vi "Read SubVIs.vi"(9 "Diagram in":refnum<class "Diagram.lvclass">) -> (3 "Diagram out":refnum<class "Diagram.lvclass">, 4 "SubVIs":refnum<class "SubVI.lvclass">[](array[class]))   [LabVIEW 2014, in "Diagram.lvclass"]
uses:
  Diagram.lvclass
  SubVI/SubVI.lvclass
  Diagram.lvclass/Diagram.ctl
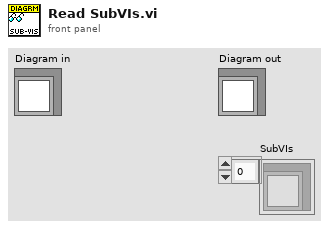
[diagram p1: front panel]
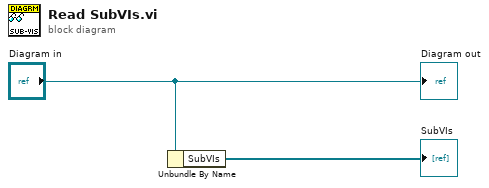
[diagram p0: block diagram]
diagram:
  n1 = Unbundle By Name("Diagram in") -> ("SubVIs"=→"SubVIs":refnum<class "SubVI.lvclass">[])
  "Diagram out" <- "Diagram in"
